vi "Custom two options Message.vi"(7 "MSG":string, 8 "Red text":string="Abortar", 11 "Green text":string="Reintentar") -> (2 "Ok?":bool)   [LabVIEW 2021]
panel:
  in  "OK 2":bool
  in  "OK":bool
  in  "Title":string
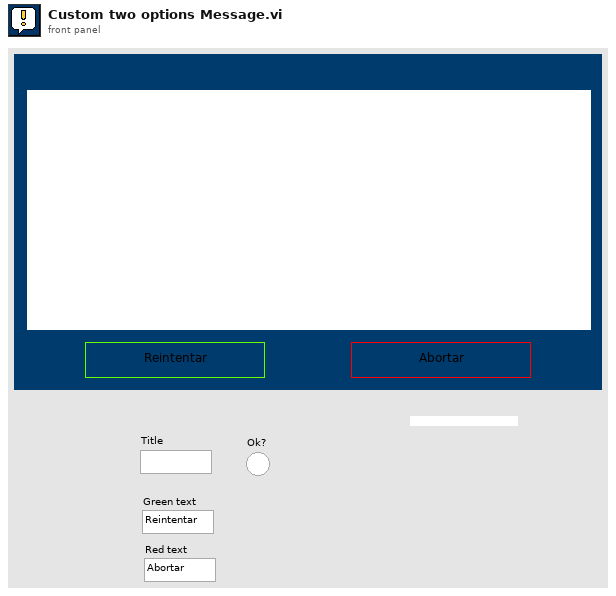
[diagram p1: front panel]
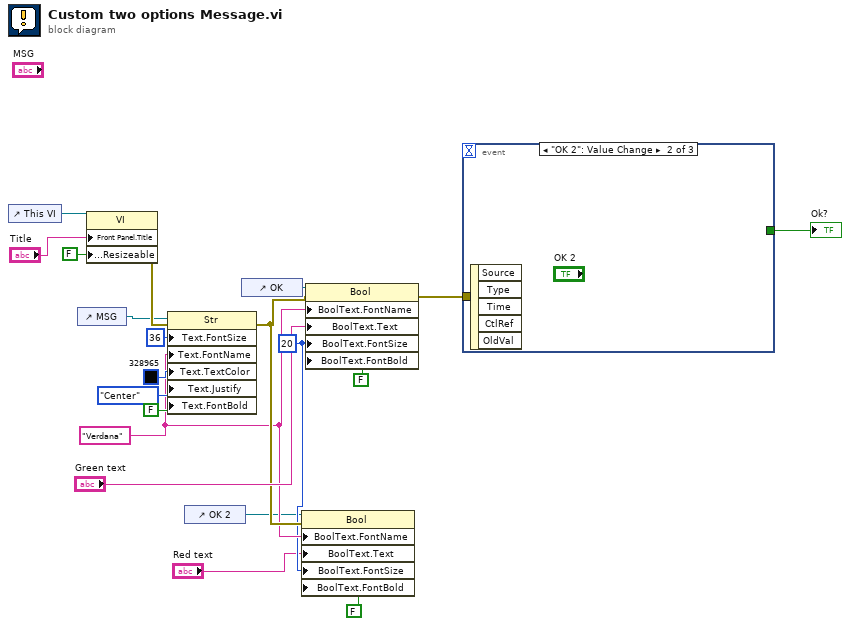
[diagram p0: block diagram]
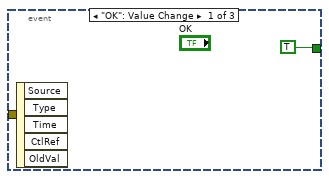
[diagram p2: hidden frame]
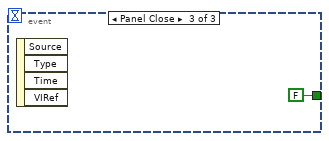
[diagram p3: hidden frame]
diagram:
  w4 = u32 20 ("Boolean Text.Font:Size")
  w5 = "Verdana" ("Text.Font:Name")
  n1 = control-ref of="This VI"() -> (w16:refnum<vi>)
  n2 = control-ref of="MSG"() -> (w9:refnum<vi>)
  n3 = property class="VI"(reference=w16, "Front Panel.Title"="Title", "Front Panel.Resizeable"=FALSE ("Front Panel Window:Resizable")) -> (error out=w14:errorcluster)  [unwired: 1 in, 1 out]
  n4 = property on="Property Node" class="Str"(reference=w9, error in=w14, "Text.FontSize"=u32 36 ("Text.Font:Size"), "Text.FontName"=w5, "Text.TextColor"=u32 328965 ("Text.Text Colors:Text Color"), "Text.Justify"=enum16{"Left", "Center", "Right"}."Center" ("Text.Justification"), "Text.FontBold"=FALSE ("Text.Font:Bold")) -> (error out=w6:errorcluster)  [unwired: 1 out]
  n5 = control-ref of="OK 2"() -> (w1:refnum<vi>)
  n6 = control-ref of="OK"() -> (w11:refnum<vi>)
  n7 = property on="Property Node" class="Bool"(reference=w1, error in=w6, "BoolText.FontName"=w5, "BoolText.Text"="Red text", "BoolText.FontSize"=w4, "BoolText.FontBold"=FALSE ("Boolean Text.Font:Bold")) -> ()  [unwired: 2 out]
  n8 = property on="Property Node" class="Bool"(reference=w11, error in=w6, "BoolText.FontName"=w5, "BoolText.Text"="Green text", "BoolText.FontSize"=w4, "BoolText.FontBold"=FALSE ("Boolean Text.Font:Bold")) -> (error out=w10:errorcluster)  [unwired: 1 out]
  n9 = event shown="[1] \"OK 2\": Value Change" {
    selector: _ -> [_ _ _]
    dyn-events: _ -> [_ _ _]
    timeout: _ -> [_ _ _]
    tunnel: [TRUE _ FALSE] -> w17
    tunnel: w10 -> [_ _ _]
    event "OK": Value Change {
      n10 = event-data() -> ()  [unwired: 6 out]
    }
    event "OK 2": Value Change {
      n11 = event-data() -> ()  [unwired: 6 out]
    }
    event Panel Close {
      n12 = event-data() -> ()  [unwired: 5 out]
    }
  }
  "Ok?" <- w17
